vi "EOL CAN_Enable_Production_Mode.vi"(8 "Error in":errorcluster, 10 "Read Session in":refnum<k21>, 11 "Write Session in":refnum<k21>) -> (0 "Error out":errorcluster, 2 "debug log":string[][](array[string]), 3 "Response Good?":bool)   [LabVIEW 2018]
uses:
  <vilib>/xnet/xnet.llb/XNET Frame CAN.ctl
  <vilib>/xnet/xnet.llb/XNET Frame Type CAN.ctl
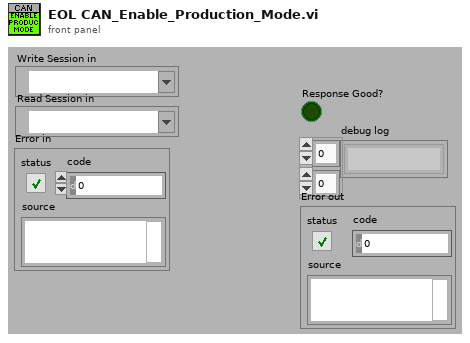
[diagram p1: front panel]
types:
  T1 = typedef "XNET Frame CAN.ctl" = cluster{"timestamp":timestamp, "payload":u8[], "identifier":u32, "type":T2, "extended?":bool, "echo?":bool}
  T2 = typedef "XNET Frame Type CAN.ctl" = u8
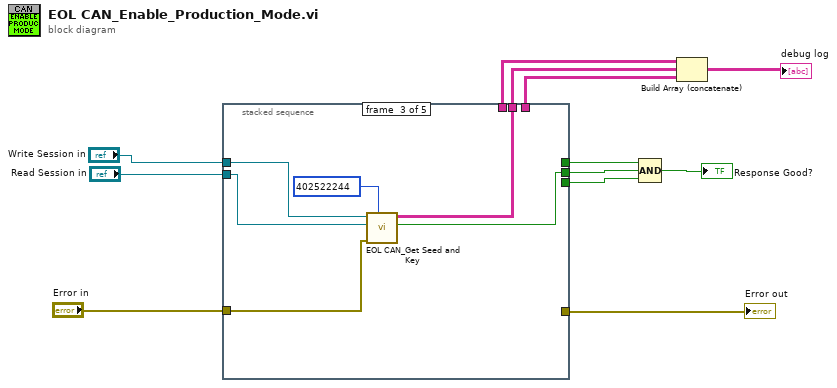
[diagram p0: block diagram]
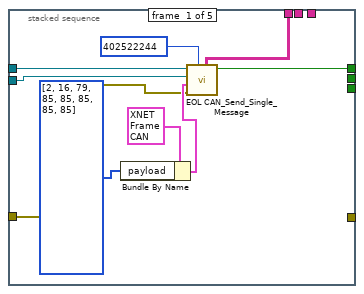
[diagram p2: hidden frame]
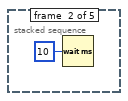
[diagram p3: hidden frame]
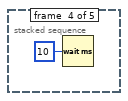
[diagram p4: hidden frame]
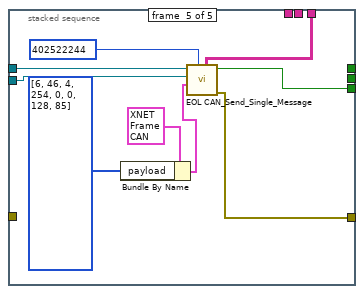
[diagram p5: hidden frame]
diagram:
  n1 = stacked-sequence {
    tunnel: [w21 _ _ _ _] -> w12
    tunnel: [w20 _ _ _ _] -> w10
    tunnel: "Write Session in" -> [w19 _ w28 _ w38]
    tunnel: "Read Session in" -> [w18 _ w27 _ w37]
    tunnel: [_ _ w26 _ _] -> w6
    tunnel: [_ _ w25 _ _] -> w5
    tunnel: [_ _ _ _ w32] -> w4
    tunnel: [_ _ _ _ w31] -> w3
    tunnel: "Error in" -> [w13 _ w23 _ _]
    tunnel: [_ _ _ _ w30] -> w1
    frame #0 {
      n2 = Bundle By Name(cluster=T1 {"timestamp"=timestamp(0 s since 1904-01-01), "payload"=[2, 39, 3, 85, 85, 85, 85, 85], "identifier"=402391172, "type"=8, "extended?"=TRUE, "echo?"=FALSE} ("Tx CAN frame"), "payload"=u8[] [2, 16, 79, 85, 85, 85, 85, 85] ("Transmit Data 2")) -> (w16:T1)
      n3 = call "EOL CAN_Send_Single_Message.vi"("Rx Arbitration Id"=u32 402522244, "Error in"=w13, "Tx CAN frame"=w16, "Read Session in"=w18, "Write Session in"=w19) -> ("Response Good?"=w21:bool, "TxRx Data"=w20:string[][])  [unwired: 2 in, 3 out]
    }
    frame #1 {
      n4 = Wait (ms)(milliseconds to wait=u32 10) -> ()  [unwired: 1 out]
    }
    frame #2 {
      n5 = call "EOL CAN_Get Seed and Key.vi"("Rx Arbitration Id"=u32 402522244, "Error in"=w23, "Read Session in"=w27, "Write Session in"=w28) -> ("Response Good?"=w25:bool, "TxRx Data"=w26:string[][])  [unwired: 5 in, 1 out]
    }
    frame #3 {
      n6 = Wait (ms)(milliseconds to wait=u32 10) -> ()  [unwired: 1 out]
    }
    frame #4 {
      n7 = Bundle By Name(cluster=T1 {"timestamp"=timestamp(0 s since 1904-01-01), "payload"=[2, 39, 3, 85, 85, 85, 85, 85], "identifier"=402391172, "type"=8, "extended?"=TRUE, "echo?"=FALSE} ("Tx CAN frame"), "payload"=u8[] [6, 46, 4, 254, 0, 0, 128, 85] ("Transmit Data 2")) -> (w36:T1)
      n8 = call "EOL CAN_Send_Single_Message.vi"("Rx Arbitration Id"=u32 402522244, "Tx CAN frame"=w36, "Read Session in"=w37, "Write Session in"=w38) -> ("Error out"=w30:errorcluster, "Response Good?"=w31:bool, "TxRx Data"=w32:string[][])  [unwired: 3 in, 2 out]
    }
  }
  "Error out" <- w1
  n9 = Compound Arithmetic op=AND(w12, w5, w3) -> (→"Response Good?":bool)
  n10 = Build Array (concatenate)(w10, w6, w4) -> (→"debug log":string[][])
